vi "movimentacao_cin_inv_bezier_2.vi"() -> ()   [LabVIEW 2017]
doc: "The myRIO Project template acquires acceleration data from the onboard accelerometer and displays the changes of acceleration values in a waveform chart."
uses:
  <vilib>/Analysis/Matrix/Datatypes/RealMatrix.ctl
  <vilib>/myRIO/Instrument Drivers/Onboard IO/PWM/typedefs/PWM Reference.ctl
  <vilib>/myRIO/Common/Instrument Driver Framework/Utilities/typedefs/myRIO Generic Hardware Reference.ctl
  <vilib>/myRIO/Common/Instrument Driver Framework/Utilities/typedefs/Hardware Version Enum.ctl
  <vilib>/myRIO/Common/Instrument Driver Framework/Utilities/typedefs/myRIO v1.0 Reference.ctl
  <vilib>/myRIO/Common/Instrument Driver Framework/Utilities/typedefs/Generic FPGA Reference.ctl
  <vilib>/myRIO/Common/Instrument Driver Framework/myRIO v1.0/PWM/typedefs/PWM Channels Enum.ctl
  <vilib>/myRIO/Instrument Drivers/Onboard IO/PWM/typedefs/PWM Configuration.ctl
  <vilib>/userdefined/High Color/nirio_resource_hc.ctl
  <vilib>/myRIO/Common/Instrument Driver Framework/myRIO v1.0/PWM/vis/myRIO v1.1 Open PWM.vi
  <vilib>/myRIO/Common/Instrument Driver Framework/Utilities/vis/Validate Channels.vi
  <vilib>/myRIO/Common/Instrument Driver Framework/myRIO v1.0/PWM/vis/myRIO v1.0 Reserve PWM.vi
  <vilib>/myRIO/Instrument Drivers/Onboard IO/PWM/vis/Set Duty Cycle and Frequency.vi
  <vilib>/myRIO/Common/Instrument Driver Framework/myRIO v1.0/PWM/vis/myRIO v1.0 Close PWM.vi
  <vilib>/myRIO/Common/Instrument Driver Framework/myRIO v1.0/PWM/vis/myRIO v1.0 Build MUX Configuration PWM.vi
  <vilib>/myRIO/Common/Instrument Driver Framework/myRIO v1.0/Resource Manager/vis/myRIO v1.0 Reserve Channel List.vi
  <vilib>/myRIO/Common/Instrument Driver Framework/myRIO v1.0/PWM/vis/myRIO v1.0 Unreserve PWM.vi
  <vilib>/myRIO/Common/Instrument Driver Framework/myRIO v1.0/Resource Manager/vis/myRIO v1.0 Create Configuration List.vi
  <vilib>/myRIO/Common/Instrument Driver Framework/myRIO v1.0/Resource Manager/vis/myRIO v1.0 Reserve Channel.vi
  <vilib>/myRIO/Common/Instrument Driver Framework/myRIO v1.0/Resource Manager/vis/myRIO v1.0 Unreserve Channel.vi
  <vilib>/myRIO/Common/Instrument Driver Framework/myRIO v1.0/Resource Manager/vis/myRIO v1.0 Unreserve Channel List.vi
  <vilib>/myRIO/Common/Instrument Driver Framework/myRIO v1.0/Resource Manager/vis/myRIO v1.0 Build Mutex Name.vi
  <vilib>/Utility/VariantDataType/GetNumericInfo.vi
  <vilib>/Utility/error.llb/Error Cluster From Error Code.vi
  <vilib>/myRIO/Common/Instrument Driver Framework/myRIO v1.0/myRIO v1.1 Open.vi
  <vilib>/myRIO/Common/Instrument Driver Framework/Utilities/vis/IO Manager.vi
  <vilib>/myRIO/Common/Instrument Driver Framework/Utilities/vis/Configuration Manager.vi
  <vilib>/myRIO/Common/Instrument Driver Framework/myRIO v1.0/Resource Manager/vis/myRIO v1.0 Configure IO.vi
  <vilib>/myRIO/Common/Instrument Driver Framework/myRIO v1.0/myRIO v1.0 Close.vi
  <vilib>/myRIO/Common/Instrument Driver Framework/myRIO v1.0/PWM/vis/myRIO v1.0 Write PWM.vi
  <vilib>/myRIO/Common/Instrument Driver Framework/myRIO v1.0/PWM/vis/myRIO v1.0 Shutdown PWM.vi
  <vilib>/myRIO/Instrument Drivers/Onboard IO/PWM/vis/myRIO PWM Open.xnode
  <vilib>/myRIO/Instrument Drivers/Onboard IO/PWM/PWM.lvlib
  <vilib>/Analysis/Matrix/NI_Matrix.lvlib
panel:
  out "iterador":u32
  out "number of rows":i32
  out "matrix":T1
  in  "Ring":u16(ring) items=["A", "B", "C"]
  out "x .and. y?":bool
  in  "OK Button":bool
  out "subarray":dbl[](array[numeric])
  out "appended array 2":dbl[](array[numeric])
  out "logical AND":bool
  out "x = y?":bool[](array[boolean])
  out "POS_E_ORIEN_HOME":dbl[](array[numeric])
  out "ANG_POSI_E_ORIEN_HOME":dbl[](array[numeric])
  out "CURRENT POSITIONS OF THE MOTORS":dbl[](array[numeric])
  in  "angulo_garra":dbl(knob) scale=-180.0..180.0
  in  "Duty Cycle Abert":dbl=0.04 format="%#_13g"
  out "Actuator 2":bool
  in  "Actuator":bool
  in  "Conveyor speed (mm/s)":dbl(slide)=200.0 step=1.0 scale=0.0..350.0
  out "indexador":i32
  out "Objeto detectado":bool
  out "Manipulando":bool
  out "Está em Home":bool
  out "Posicao_desejada":bool
  in  "Home":bool
  in  "error in (no error)":errorcluster
  in  "PARAR":bool
  in  "POSITION VECTOR":dbl[](array[numeric])
  # "ROTINA DE CONTROLE DO PROTÓTIPO DE FMS"
  # "COMANDO DE POSIÇÃO\nATUAL DOS MOTORES"
  # "OPERATION STATUS"
  # "ÂNGULOS DE JUNTAS"
  # "THETA 1"
  # "MOTOR 1"
  # "HOME"
  # "THETA 2"
  # "MOTOR 2"
  # "DESIRED POSITION"
  # "THETA 3"
  # "MOTOR 3"
  # "OBJECT DETECTED"
  # "THETA 4"
  # "MOTOR 4"
  # "MANIPULATING"
  # "THETA 5"
  # "MOTOR 5"
  # "ACTUATOR"
  # "MOTOR 6"
  # "VELOCIDADE DA ESTEIRA (mm/s)"
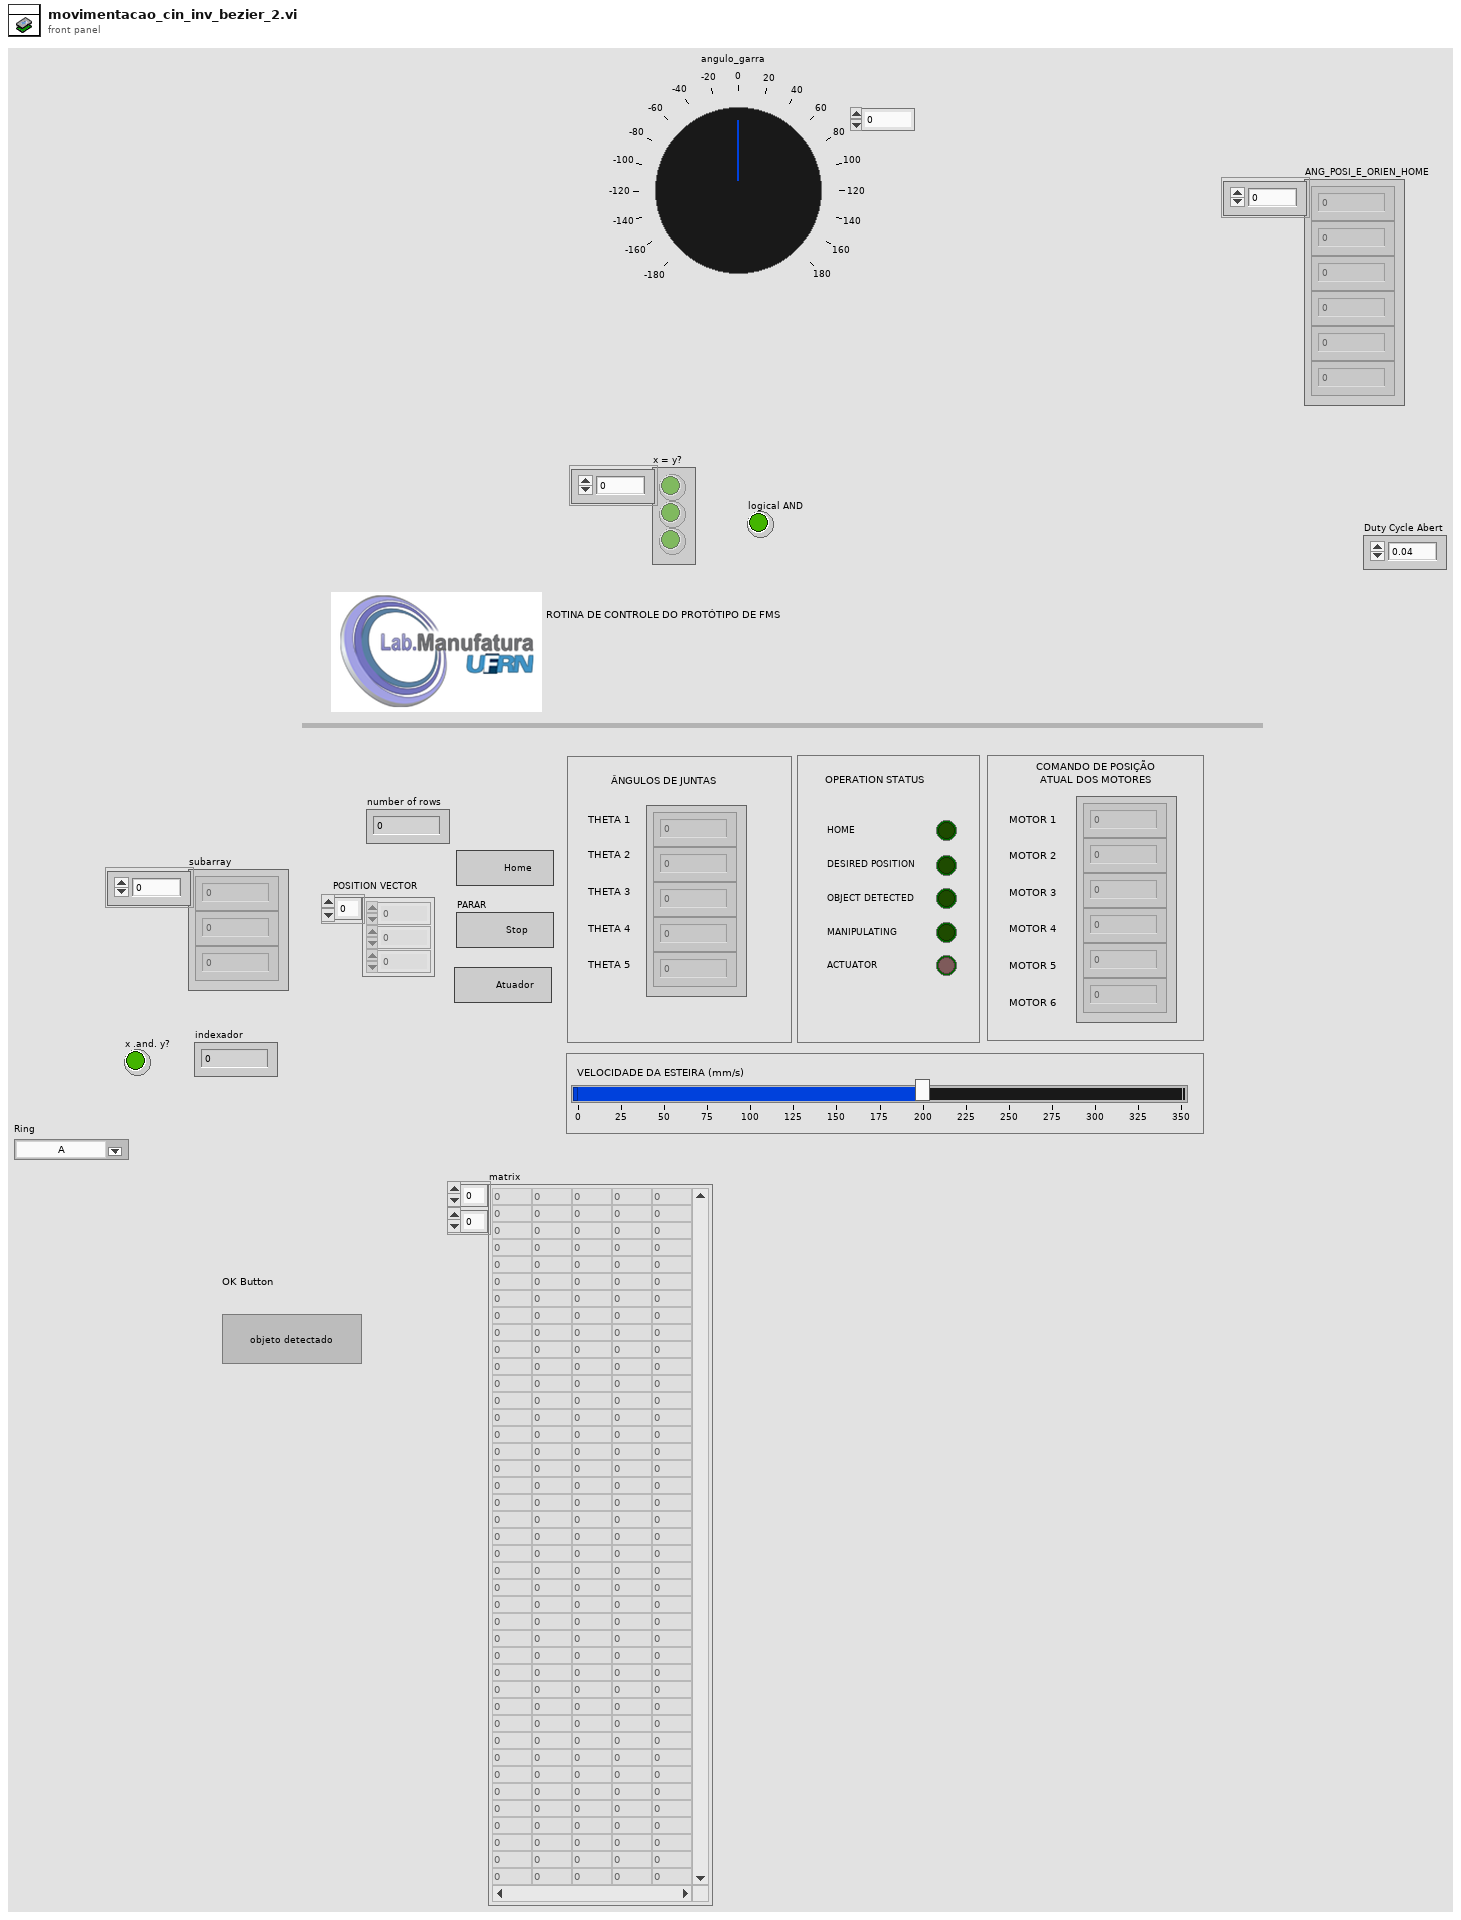
[diagram p1: front panel]
types:
  T1 = typedef "NI_Matrix.lvlib/RealMatrix.ctl" = dbl[][]
  T2 = cluster{"theta 1":dbl, "theta 2":dbl, "theta 3":dbl, "theta5":dbl, "theta4":dbl}
  T3 = typedef "nirio_resource_hc.ctl" = tag
  T4 = typedef "Hardware Version Enum.ctl" = enum16{"Unknown", "myRIO-1900", "myRIO-1950", "roboRIO", "NI ELVIS RIO CM"}
  T5 = typedef "PWM.lvlib/PWM Reference.ctl" = cluster{"myRIO Reference":T6, "PWM Channels Enum":T9, "PWM Configuration":T10}
  T6 = typedef "myRIO Generic Hardware Reference.ctl" = cluster{"myRIO Model":T4, "myRIO Hardware Reference":T7}
  T7 = typedef "myRIO v1.0 Reference.ctl" = cluster{"Generic FPGA Reference":T8, "Allow multiple opens":bool}
  T8 = typedef "Generic FPGA Reference.ctl" = refnum<k20>
  T9 = typedef "PWM Channels Enum.ctl" = enum16{"Not Connected", "C/PWM0", "C/PWM1", "A/PWM0", "A/PWM1", "A/PWM2", "B/PWM0", "B/PWM1", "B/PWM2", "PWM/PWM0", "PWM/PWM1", "PWM/PWM2", "PWM/PWM3", "PWM/PWM4", "PWM/PWM5", "PWM/PWM6", "PWM/PWM7", "PWM/PWM8", "PWM/PWM9"}
  T10 = typedef "PWM.lvlib/PWM Configuration.ctl" = cluster{"Frequency":dbl, "Duty Cycle":dbl}
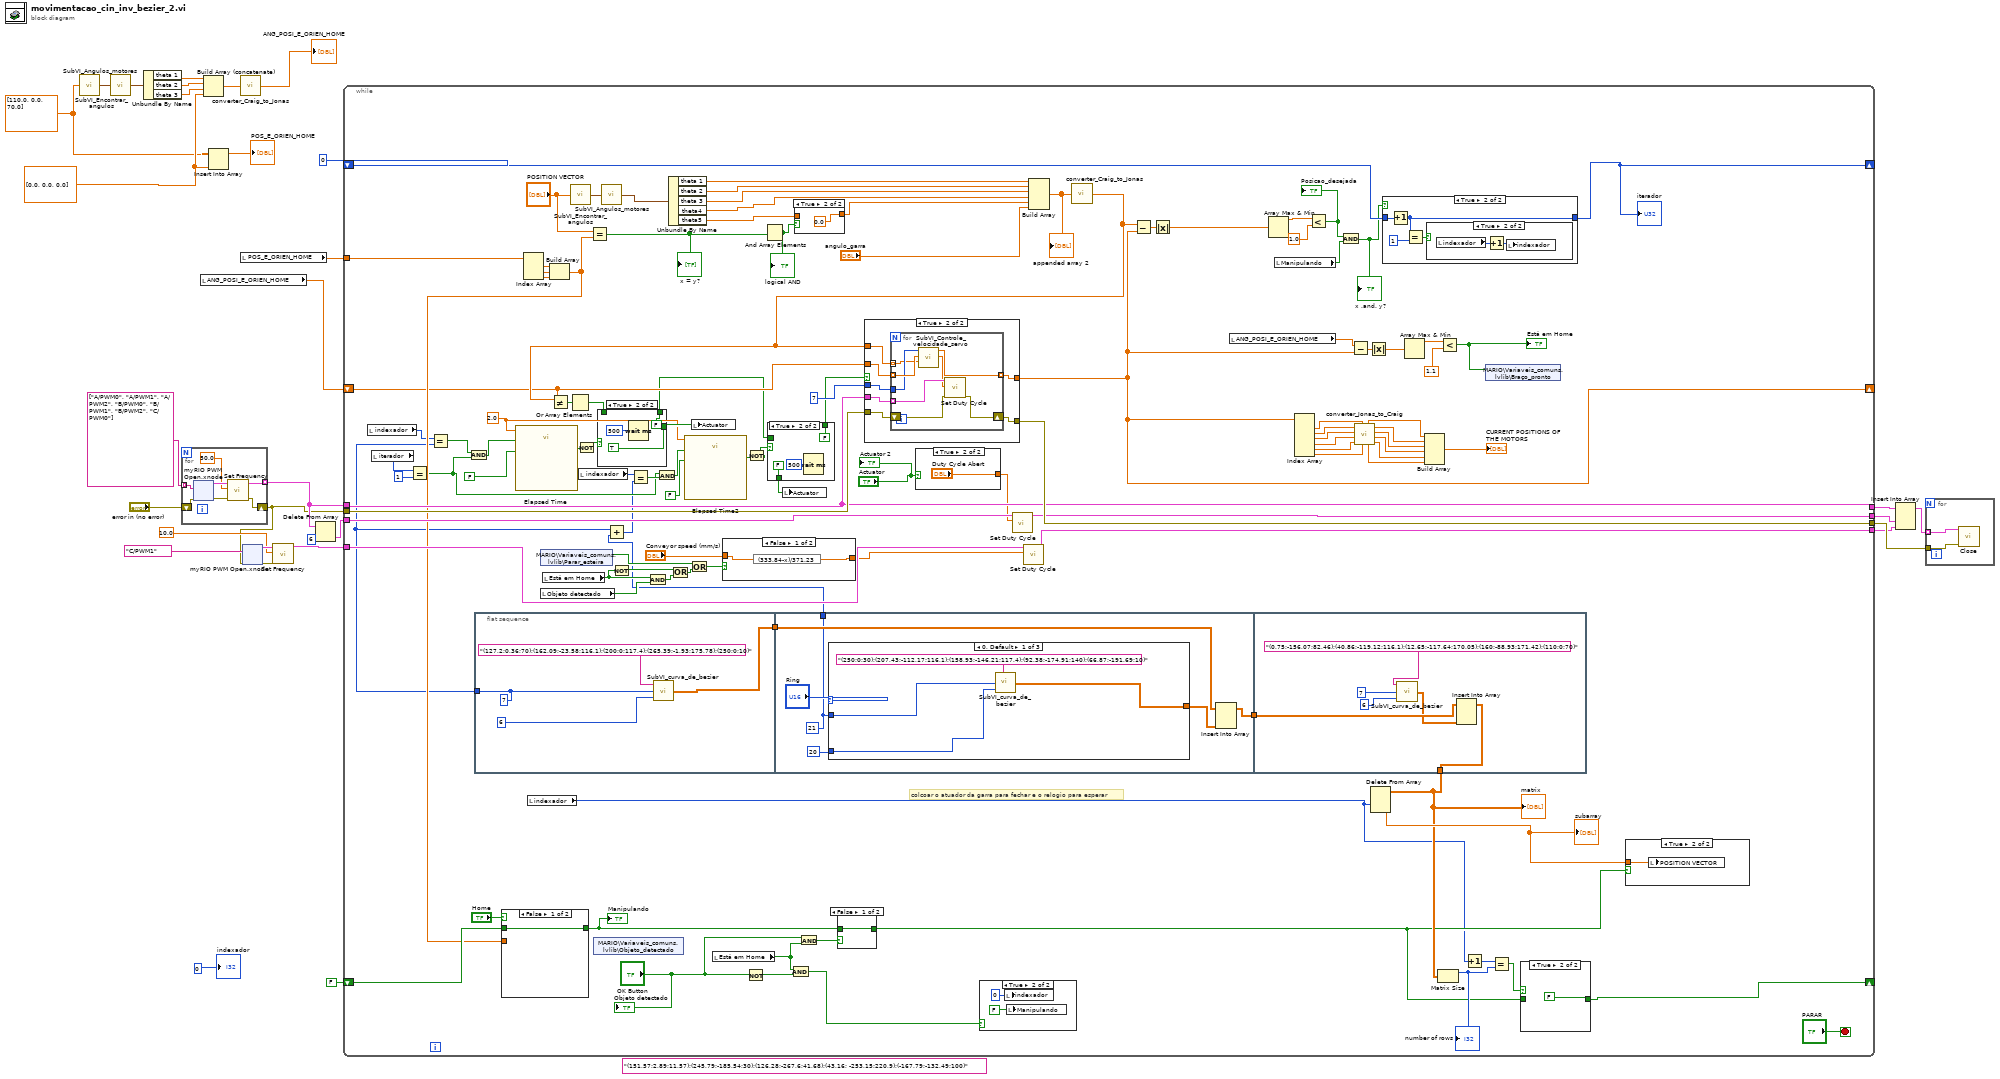
[diagram p0: block diagram]
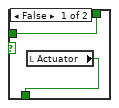
[diagram p2: hidden frame]
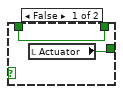
[diagram p3: hidden frame]
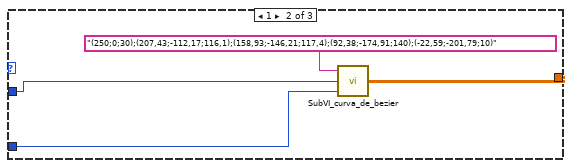
[diagram p5: hidden frame]
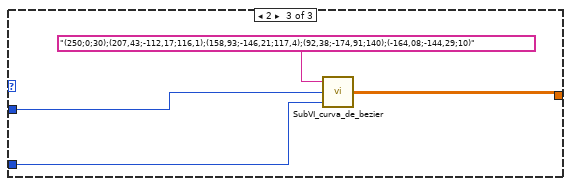
[diagram p6: hidden frame]
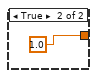
[diagram p7: hidden frame]
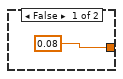
[diagram p8: hidden frame]
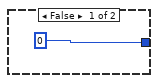
[diagram p11: hidden frame]
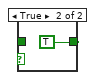
[diagram p14: hidden frame]
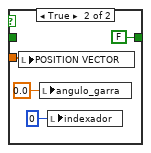
[diagram p15: hidden frame]
diagram:
  (unwired) "(151,57;2,89;11,57);(245,79;-185,54;30);(126,28;-267,6;41,68);(43,16; -253,15;220,9);(-167,79;-132,49;100)" ("String 2")
  w8 = dbl[] [0.0, 0.0, 0.0] ("vetor_P")
  w3 = dbl[] [110.0, 0.0, 70.0] ("vetor_P")
  n1 = call "SubVI_Encontrar_angulos.vi"("vetor_P"=w3) -> ("ângulos de Juntas"=w2:T2)
  n2 = call "SubVI_Angulos_motores.vi"("input cluster"=w2) -> ("output cluster"=w1:T2)
  n3 = Unbundle By Name(w1) -> ("theta 1"=w12:dbl, "theta 2"=w11:dbl, "theta 3"=w10:dbl)
  n4 = for {
    tunnel: tag[] ["A/PWM0", "A/PWM1", "A/PWM2", "B/PWM0", "B/PWM1", "B/PWM2", "C/PWM0"] -> [w35] mode=indexing
    tunnel: [w34] -> w25 mode=indexing
    shift-right: [w33] -> w14
    shift-left: "error in (no error)" -> [w32]
    n5 = xnode ("myRIO PWM Open.xnode")("error in (no error)"=w32, "Channel Name"=w35) -> ("error out"=w36:errorcluster, "PWM Ref Out"=w38:T5)  [unwired: 1 in]
    n6 = call <vilib>:"Set Frequency.vi"("error in (no error)"=w36, "Frequency [Hz]"=50.0, "PWM Ref In"=w38) -> ("error out"=w33:errorcluster, "PWM Ref Out"=w34:T5)  [unwired: 6 in]
  }
  n7 = local read "ANG_POSI_E_ORIEN_HOME"() -> (w9:dbl[])
  n8 = Build Array (concatenate)(w12, w11, w10, w8) -> (w5:dbl[])
  n9 = Insert Into Array(array=w3, new element=w8) -> (→"POS_E_ORIEN_HOME":dbl[])  [unwired: 1 in]
  n10 = call "converter_Craig_to_Jonas.vi"("array"=w5) -> ("appended array"=→"ANG_POSI_E_ORIEN_HOME":dbl[])
  n11 = local read "POS_E_ORIEN_HOME"() -> (w6:dbl[])
  n12 = xnode "myRIO PWM Open.xnode"("error in (no error)"=w14, "Channel Name"=tag "C/PWM1") -> ("error out"=w18:errorcluster, "PWM Ref Out"=w19:T5)  [unwired: 1 in]
  n13 = call <vilib>:"Set Frequency.vi"("error in (no error)"=w18, "Frequency [Hz]"=10.0, "PWM Ref In"=w19) -> ("PWM Ref Out"=w15:T5)  [unwired: 6 in, 1 out]
  n14 = Delete From Array(array=w25, index=6) -> (deleted portion=w23:T5)  [unwired: 1 in, 1 out]
  n15 = while {
    tunnel: [w165] -> w31
    shift-right: [w97] -> _
    shift-left: w9 -> [w89]
    tunnel: w14 -> [w163]
    tunnel: w25 -> [w162]
    tunnel: [w162] -> w22
    shift-right: [w82] -> _
    shift-left: FALSE -> [w146]
    shift-right: [w155] -> _
    shift-left: u32 0 ("ms to wait (braço)") -> [w154]
    tunnel: w23 -> [w141]
    tunnel: [w140] -> w21
    tunnel: w15 -> [w138]
    tunnel: [w134] -> w13
    tunnel: w6 -> [w104]
    stop <- "PARAR" stop-if-true
    w64 = 2.0 ("Time Target (s)")
    # "colcoar o atuador da garra para fechar e o relogio para esperar"
    n16 = local read "indexador"() -> (w76:i32)
    n17 = local read "iterador"() -> (w78:u32)
    n18 = Equal?(x=w78, y=u32 1) -> (x = y?=w66:bool)
    n19 = Equal?(x=w76, y=w55) -> (x = y?=w69:bool)
    n20 = And(x=w69, y=w66) -> (x .and. y?=w75:bool)
    n21 = flat-sequence {
      tunnel: [w180] -> w85
      tunnel: [w178] -> w55
      tunnel: w85 -> [w185]
      tunnel: [w186] -> w84
      tunnel: [w182] -> w56
      tunnel: [w200] -> w83
      tunnel: w84 -> [w202]
      frame #0 {
        w178 = i64 7 ("número de pontos que a matriz deve retornar (nº de divisões + 1)")
        n22 = call "SubVI_curva_de_bezier.vi"("Nº de divisões da curva de Bézier (padrão: 20 divisões = 21 pontos)"=6, "número de pontos que a matriz deve retornar (padrão: nº de divisões + 1)"=w178, "String in"="(127,2;0,36;70);(162,09;-23,58;116,1);(200;0;117,4);(265,39;-1,93;175,78);(250;0;10)" ("Esteira")) -> ("matrix"=w180:T1)
      }
      frame #1 {
        w182 = i64 21 ("número de pontos que a matriz deve retornar (nº de divisões + 1)")
        n23 = case shown="0, Default" "Ring" {
          tunnel: [w191 w195 w199] -> w184
          tunnel: w182 -> [w189 w193 w197]
          tunnel: 20 ("Nº de divisões da curva de Bézier (padrão: 20 divisões = 21 pontos)") -> [w188 w192 w196]
          frame 0, Default {
            n24 = call "SubVI_curva_de_bezier.vi"("Nº de divisões da curva de Bézier (padrão: 20 divisões = 21 pontos)"=w188, "número de pontos que a matriz deve retornar (padrão: nº de divisões + 1)"=w189, "String in"="(250;0;30);(207,43;-112,17;116,1);(158,93;-146,21;117,4);(92,38;-174,91;140);(66,87;-191,69;10)" ("Esteira")) -> ("matrix"=w191:T1)
          }
          frame 1 {
            n25 = call "SubVI_curva_de_bezier.vi"("Nº de divisões da curva de Bézier (padrão: 20 divisões = 21 pontos)"=w192, "número de pontos que a matriz deve retornar (padrão: nº de divisões + 1)"=w193, "String in"="(250;0;30);(207,43;-112,17;116,1);(158,93;-146,21;117,4);(92,38;-174,91;140);(-22,59;-201,79;10)" ("Esteira")) -> ("matrix"=w195:T1)
          }
          frame 2 {
            n26 = call "SubVI_curva_de_bezier.vi"("Nº de divisões da curva de Bézier (padrão: 20 divisões = 21 pontos)"=w196, "número de pontos que a matriz deve retornar (padrão: nº de divisões + 1)"=w197, "String in"="(250;0;30);(207,43;-112,17;116,1);(158,93;-146,21;117,4);(92,38;-174,91;140);(-164,08;-144,29;10)" ("Esteira")) -> ("matrix"=w199:T1)
          }
        }
        n27 = Insert Into Array(array=w185, new element=w184) -> (w186:T1)  [unwired: 2 in]
      }
      frame #2 {
        n28 = call "SubVI_curva_de_bezier.vi"("Nº de divisões da curva de Bézier (padrão: 20 divisões = 21 pontos)"=6, "número de pontos que a matriz deve retornar (padrão: nº de divisões + 1)"=i64 7 ("número de pontos que a matriz deve retornar (nº de divisões + 1)"), "String in"="(0,75;-156,07;82,46);(40,86;-119,12;116,1);(12,65;-117,64;170,05);(160;-88,93;171,42);(110;0;70)" ("Esteira")) -> ("matrix"=w201:T1)
        n29 = Insert Into Array(array=w202, new element=w201) -> (w200:T1)  [unwired: 2 in]
      }
    }
    n30 = call "Elapsed Time"("Time Target (s)"=w64, "Reset"=w75, "Auto Reset"=FALSE) -> ("Time has Elapsed"=w73:bool)  [unwired: 9 in, 7 out]
    n31 = Index Array(array=w104) -> (element #1=w107:dbl, element #2=w106:dbl, element #3=w105:dbl)  [unwired: 3 in]
    n32 = local read "indexador"() -> (w79:i32)
    n33 = shared-variable "MARIO\\Variaveis_comuns.lvlib\\Parar_esteira"() -> (w133:bool)  [unwired: 1 in, 1 out]
    n34 = local read "Objeto detectado"() -> (w131:bool)
    n35 = local read "Está em Home"() -> (w128:bool)
    n36 = Build Array(w107, w106, w105) -> (w103:dbl[])
    n37 = case shown="False" "Home" {
      tunnel: w103 -> [_ w230]
      tunnel: w146 -> [w226 _]
      tunnel: [w226 FALSE ("Manipulando")] -> w96
      frame False {
      }
      frame True {
        n38 = local write "POSITION VECTOR"(w230) -> ()
        n39 = local write "angulo_garra"(0.0 ("angulo_garra")) -> ()
        n40 = local write "indexador"(0 ("indexador")) -> ()
      }
    }
    "Manipulando" <- w96
    n41 = call "SubVI_Encontrar_angulos.vi"("vetor_P"="POSITION VECTOR") -> ("ângulos de Juntas"=w94:T2)
    n42 = Not(x=w73) -> (.not. x?=w72:bool)
    n43 = local read "indexador"() -> (w68:i32)
    n44 = Equal?(x="POSITION VECTOR", y=w103) -> (x = y?=w144:bool[])
    "x = y?" <- w144
    n45 = shared-variable "MARIO\\Variaveis_comuns.lvlib\\Objeto_detectado"() -> ()  [unwired: 1 in, 2 out]
    n46 = call "SubVI_Angulos_motores.vi"("input cluster"=w94) -> ("output cluster"=w93:T2)
    n47 = Add(x=w55, y=w56) -> (x+y=w57:i64)
    n48 = Not(x=w128) -> (.not. x?=w129:bool)
    n49 = Equal?(x=w68, y=w57) -> (x = y?=w67:bool)
    n50 = And(x=w128, y=w131) -> (x .and. y?=w130:bool)
    n51 = And(x=w66, y=w67) -> (x .and. y?=w65:bool)
    n52 = Unbundle By Name(w93) -> ("theta 1"=w113:dbl, "theta 2"=w112:dbl, "theta 3"=w111:dbl, "theta4"=w92:dbl, "theta5"=w91:dbl)
    n53 = Or(x=w129, y=w130) -> (x .or. y?=w127:bool)
    n54 = call "Elapsed Time2"("Time Target (s)"=w64, "Reset"=w65, "Auto Reset"=FALSE) -> ("Time has Elapsed"=w63:bool)  [unwired: 9 in, 7 out]
    n55 = Or(x=w133, y=w127) -> (x .or. y?=w135:bool)
    n56 = local read "Está em Home"() -> (w100:bool)
    n57 = case shown="False" w135 {
      tunnel: [w207 1.0 ("Duty Cycle")] -> w137
      tunnel: "Conveyor speed (mm/s)" -> [w206 _]
      frame False {
        n58 = expression code="(333.84-x)/371.23"(w206) -> (w207:dbl)
      }
      frame True {
      }
    }
    n59 = Not(x="OK Button") -> (.not. x?=w99:bool)
    n60 = Not(x=w63) -> (.not. x?=w62:bool)
    n61 = And Array Elements(Boolean array=w144) -> (logical AND=w143:bool)
    "logical AND" <- w143
    n62 = And(x=w100, y=w99) -> (x .and. y?=w151:bool)
    n63 = case shown="True" w143 {
      tunnel: [w211 0.0 ("theta5")] -> w110
      tunnel: w91 -> [w211 _]
      frame False {
      }
      frame True {
      }
    }
    n64 = And(x="OK Button", y=w100) -> (x .and. y?=w157:bool)
    n65 = case shown="False" w157 {
      tunnel: [w224 TRUE] -> w80
      tunnel: w96 -> [w224 _]
      frame False {
      }
      frame True {
      }
    }
    n66 = case shown="True" "Actuator" {
      tunnel: [0.08 ("Duty Cycle Abert") "Duty Cycle Abert"] -> w139
      frame False {
      }
      frame True {
      }
    }
    n67 = case shown="True" w151 {
      frame False {
      }
      frame True {
        n68 = local write "indexador"(0 ("indexador")) -> ()
        n69 = local write "Manipulando"(FALSE ("Manipulando")) -> ()
      }
    }
    n70 = call <vilib>:"Set Duty Cycle.vi"("Duty Cycle"=w139, "PWM Ref In"=w141) -> ("PWM Ref Out"=w140:T5)  [unwired: 7 in, 1 out]
    n71 = call <vilib>:"Set Duty Cycle.vi"("Duty Cycle"=w137, "PWM Ref In"=w138) -> ("PWM Ref Out"=w134:T5)  [unwired: 7 in, 1 out]
    n72 = Build Array(w113, w112, w111, w92, w110, "angulo_garra") -> (w109:dbl[])
    "appended array 2" <- w109
    n73 = call "converter_Craig_to_Jonas.vi"("array"=w109) -> ("appended array"=w102:dbl[])
    n74 = Not Equal?(x=w102, y=w89) -> (x != y?=w161:bool[])
    n75 = Or Array Elements(Boolean array=w161) -> (logical OR=w71:bool)
    n76 = case shown="True" w72 {
      tunnel: [w173 FALSE] -> w60
      tunnel: w71 -> [w173 _]
      tunnel: [w172 TRUE ("Actuator")] -> w70
      frame False {
        n77 = local read "Actuator"() -> (w172:bool)
      }
      frame True {
        n78 = Wait (ms)(milliseconds to wait=u32 500) -> ()  [unwired: 1 out]
      }
    }
    n79 = local write "Actuator"(w70) -> ()
    n80 = case shown="True" w62 {
      tunnel: [w168 FALSE ("Actuator")] -> w61
      tunnel: w60 -> [w167 _]
      tunnel: [w167 FALSE] -> w59
      frame False {
        n81 = local read "Actuator"() -> (w168:bool)
      }
      frame True {
        n82 = Wait (ms)(milliseconds to wait=u32 500) -> ()  [unwired: 1 out]
      }
    }
    n83 = local write "Actuator"(w61) -> ()
    n84 = case shown="True" w59 {
      tunnel: [w231 w239] -> w165
      tunnel: w163 -> [w231 w238]
      tunnel: w162 -> [_ w237]
      tunnel: w89 -> [w232 w236]
      tunnel: [w232 w234] -> w97
      tunnel: u32 7 ("ms to wait (braço)") -> [_ w235]
      tunnel: w102 -> [_ w233]
      frame False {
      }
      frame True {
        n85 = for {
          tunnel: w237 -> [w245] mode=indexing
          tunnel: w236 -> [w244] mode=indexing
          tunnel: w235 -> [w242]
          tunnel: [w241] -> w234 mode=indexing
          tunnel: w233 -> [w240] mode=indexing
          shift-right: [w247] -> w239
          shift-left: w238 -> [w246]
          n86 = call "SubVI_Controle_velocidade_servo.vi"("Posição Desejada"=w240, "Posição"=w244, "milliseconds to wait"=w242) -> ("Duty Cycle"=w243:dbl, "Posição"=w241:dbl)  [unwired: 7 in]
          n87 = call <vilib>:"Set Duty Cycle.vi"("error in (no error)"=w246, "Duty Cycle"=w243, "PWM Ref In"=w245) -> ("error out"=w247:errorcluster)  [unwired: 6 in, 1 out]
        }
      }
    }
    n88 = Subtract(x=w102, y=w97) -> (x-y=w160:dbl[])
    n89 = Absolute Value(x=w160) -> (abs(x)=w159:dbl[])
    n90 = local read "ANG_POSI_E_ORIEN_HOME"() -> (w108:dbl[])
    n91 = Array Max & Min(array=w159) -> (max value=w101:dbl)  [unwired: 3 out]
    n92 = local read "Manipulando"() -> (w153:bool)
    n93 = Index Array(array=w97) -> (element #1=w126:dbl, element #2=w125:dbl, element #3=w124:dbl, element #4=w123:dbl, element #5=w122:dbl, element #6=w121:dbl)  [unwired: 6 in]
    n94 = Less?(x=w101, y=1.0) -> (x < y?=w98:bool)
    "Posicao_desejada" <- w98
    n95 = And(x=w98, y=w153) -> (x .and. y?=w152:bool)
    "x .and. y?" <- w152
    n96 = Subtract(x=w108, y=w97) -> (x-y=w150:dbl[])
    n97 = call "converter_Jonas_to_Craig.vi"("theta6Jonas"=w121, "theta1Jonas"=w126, "theta5Jonas"=w122, "theta4Jonas"=w123, "theta3Jonas"=w124, "theta2Jonas"=w125) -> ("theta5Craig"=w116:dbl, "theta4Craig"=w117:dbl, "theta3Craig"=w118:dbl, "theta2Craig"=w119:dbl, "theta6Craig"=w115:dbl, "theta1Craig"=w120:dbl)
    n98 = Absolute Value(x=w150) -> (abs(x)=w149:dbl[])
    n99 = Delete From Array(array=w83, index (row)=w79) -> (deleted portion=w88:dbl[])  [unwired: 2 in, 1 out]
    "subarray" <- w88
    n100 = case shown="True" w152 {
      tunnel: w154 -> [_ w219]
      tunnel: [u32 0 ("ms to wait (braço)") w218] -> w155
      frame False {
      }
      frame True {
        n101 = Increment(x=w219) -> (x+1=w218:u32)
        n102 = Equal?(x=w218, y=u32 1) -> (x = y?=w216:bool)
        n103 = case shown="True" w216 {
          frame False {
          }
          frame True {
            n104 = local read "indexador"() -> (w221:i32)
            n105 = Increment(x=w221) -> (x+1=w220:i32)
            n106 = local write "indexador"(w220) -> ()
          }
        }
      }
    }
    "iterador" <- w155
    n107 = Array Max & Min(array=w149) -> (max value=w148:dbl)  [unwired: 3 out]
    n108 = Build Array(w120, w119, w118, w117, w116, w115) -> (→"CURRENT POSITIONS OF THE MOTORS":dbl[])
    n109 = Matrix Size(0:w83) -> (1:w87:i32)  [unwired: 1 out]
    "number of rows" <- w87
    n110 = Less?(x=w148, y=1.1) -> (x < y?=w132:bool)
    "Está em Home" <- w132
    n111 = Increment(x=w79) -> (x+1=w81:i32)
    n112 = shared-variable "MARIO\\Variaveis_comuns.lvlib\\Braço_pronto"(w132) -> ()  [unwired: 1 in, 1 out]
    n113 = Equal?(x=w81, y=w87) -> (x = y?=w145:bool)
    n114 = case shown="True" w145 {
      tunnel: [w213 FALSE ("Manipulando")] -> w82
      tunnel: w80 -> [w213 _]
      frame False {
      }
      frame True {
      }
    }
    n115 = case shown="True" w80 {
      tunnel: w88 -> [_ w177]
      frame False {
      }
      frame True {
        n116 = local write "POSITION VECTOR"(w177) -> ()
      }
    }
    "Objeto detectado" <- "OK Button"
    "Actuator 2" <- "Actuator"
    "matrix" <- w83
  }
  n117 = Insert Into Array(array=w22, new element #1=w21, new element #2=w13) -> (w20:T5[])  [unwired: 1 in]
  n118 = for {
    tunnel: w31 -> [w249]
    tunnel: w20 -> [w248] mode=indexing
    n119 = call <vilib>:"Close.vi"("error in (no error)"=w249, "PWM Ref In"=w248) -> ()  [unwired: 9 in, 1 out]
  }
  "indexador" <- 0
